vi "Calibration Helper.vi"(6 "Std Devs":cluster{"H":dbl, "S":dbl, "V":dbl}={"H"=4.0, "S"=6.0, "V"=4.0}, 8 "Color Mode":u16(ring)=2 items=["RGB", "HSL", "HSV", "HSI", "CIE L*a*b*", "CIE XYZ"], 9 "Color Components":T1={"Hue"={110.0, 142.0}, "Sat"={138.0, 255.0}, "Val"={139.0, 198.0}} {"Val" scale=0.0..255.0; "Sat" scale=0.0..255.0; "Hue" scale=0.0..255.0 scale format="%#_3g"}, 10 "Image":T2, 11 "Image Ctl Refnum":refnum<vi>) -> (2 "Changed":bool, 3 "output color":T3)   [LabVIEW 2025]
doc: "Process mouse clicks on the image control to compute a color range that describes the highlighted region. The range is based on the center and standard deviation returned by a histogram of the region."
uses:
  <vilib>/vision/Image Controls.llb/IMAQ Image.ctl
  <vilib>/vision/NI_Vision_Development_Module.lvlib
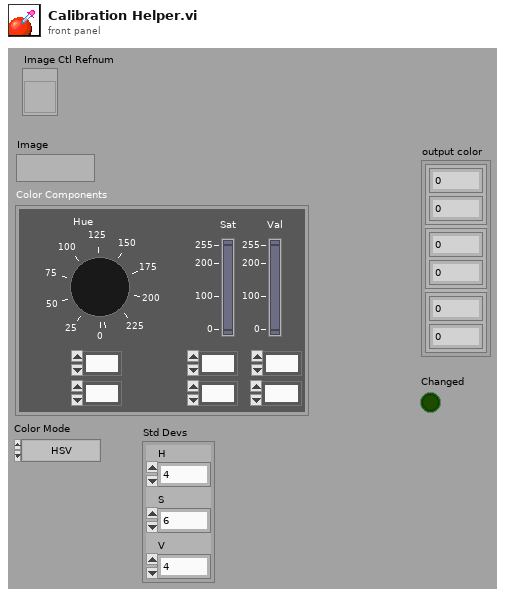
[diagram p1: front panel]
types:
  T1 = cluster{"Hue":cluster{dbl, dbl}, "Sat":cluster{dbl, dbl}, "Val":cluster{dbl, dbl}}
  T2 = typedef "IMAQ Image.ctl" = refnum<image>
  T3 = cluster{cluster{dbl, dbl}, cluster{dbl, dbl}, cluster{dbl, dbl}}
  T4 = typedef "Image Type" = u32
  T5 = cluster{"Global Rectangle":i32[], "Contours":cluster{"Contour Type":u32, "ROI Type":u32, "Points":i32[]}[]}
  T6 = cluster{"histogram":u32[], "Minimal Value":sgl, "Maximal Value":sgl, "Starting Value":sgl, "Interval Width":sgl, "Mean Value":sgl, "Standard  Variation":sgl, "Area (pixels)":i32}
  T7 = cluster{"histogram":u32[], "Minimal Value":sgl, "Maximal Value":sgl, "Starting Value":sgl, "Interval Width":sgl, "Mean Value":sgl, "Standard  Variation":sgl, "Area (pixels)":i32}[]
  T8 = cluster{"[0]":cluster{dbl, dbl}, "[1]":cluster{dbl, dbl}, "[2]":cluster{dbl, dbl}}
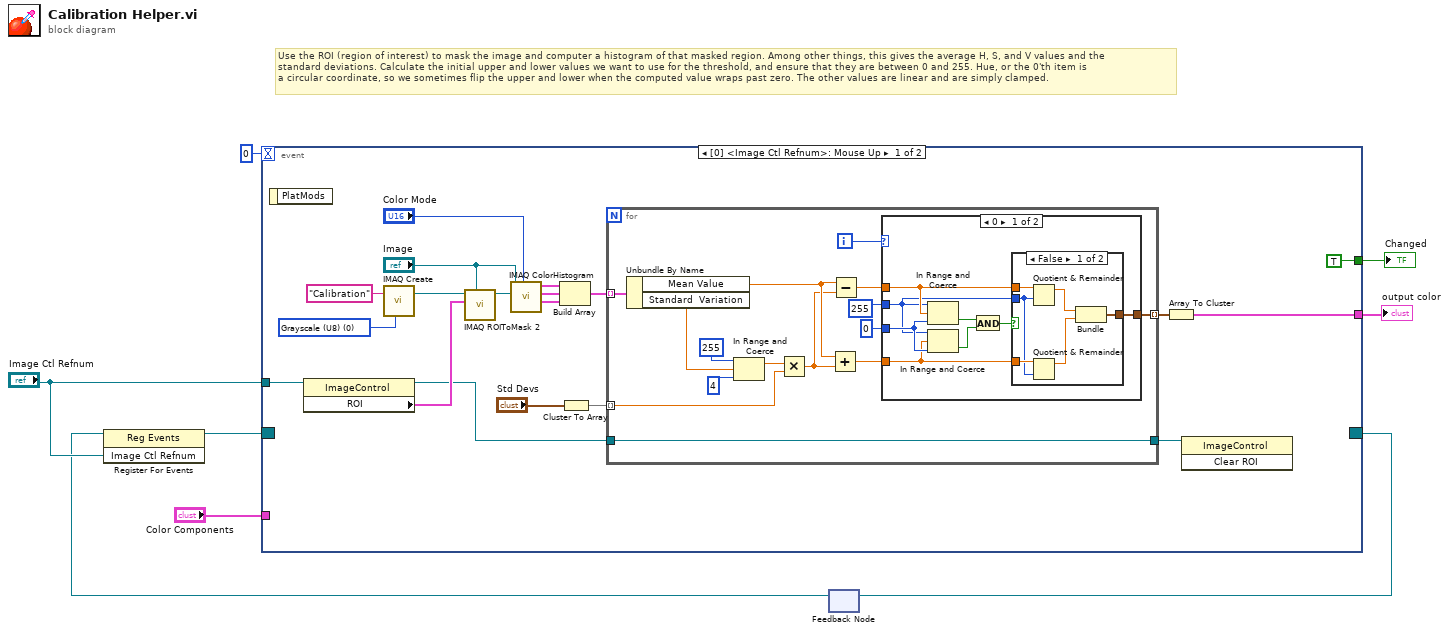
[diagram p0: block diagram]
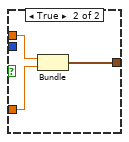
[diagram p2: hidden frame]
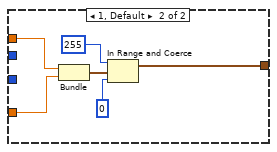
[diagram p3: hidden frame]
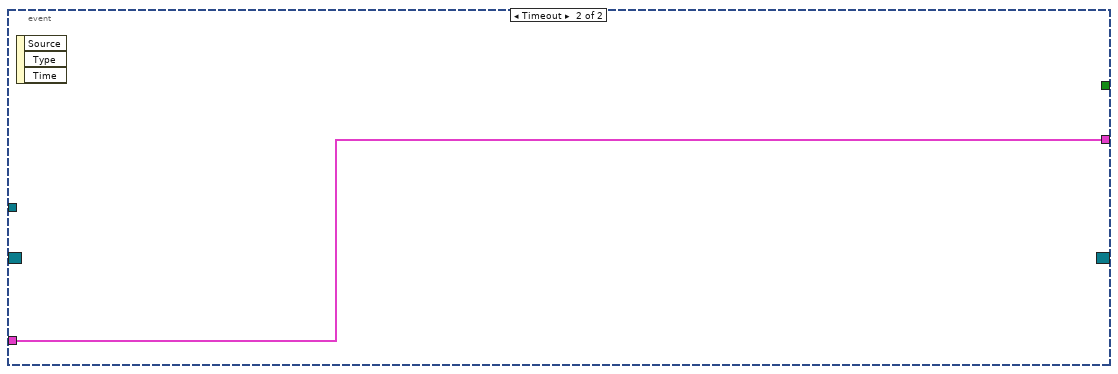
[diagram p4: hidden frame]
diagram:
  # "Use the ROI (region of interest) to mask the image and computer a histogram of that masked region. Among other things, this gives the average H, S, and V values and the\nstandard deviations. Calculate the initial upper and lower values we want to use for the threshold, and ensure that they are between 0 and 255. Hue, or the 0'th item is\na circular coordinate, so we sometimes flip the upper and lower when the computed value wraps past zero. The other values are linear and are simply clamped."
  n1 = feedback #1() -> (w2:refnum<event-registration>)  [unwired: 1 in]
  n2 = register-events(reference=w2, "Image Ctl Refnum") -> (reference out=w6:refnum<event-registration>)  [unwired: 1 in, 1 out]
  n3 = event shown="[0] <Image Ctl Refnum>: Mouse Up" {
    selector: w6 -> [_ _]
    dyn-events: [_ _] -> w3
    timeout: 0 -> [_ _]
    tunnel: "Image Ctl Refnum" -> [w14 _]
    tunnel: "Color Components" -> [_ w66]
    tunnel: [w10 w66] -> w4
    tunnel: [TRUE _] -> w1
    event Mouse Up {
      w27 = T4 0 items=["Grayscale (U8)", "Grayscale (I16)", "Grayscale (SGL)", "Complex (CSG)", "RGB (U32)", "HSL (U32)", "RGB (U64)", "Grayscale (U16)"] ("Image Type")
      n4 = event-data() -> ()  [unwired: 1 in, 1 out]
      n5 = property on="Property Node" class="ImageControl"(reference=w14) -> (reference out=w11:refnum<vi>, "ROI"=w13:T5)  [unwired: 1 in, 1 out]
      n6 = call "IMAQ Create"("Image Name"="Calibration", "Image Type"=w27) -> ("New Image"=w24:T2)  [unwired: 3 in, 1 out]
      n7 = call "IMAQ ROIToMask 2"("Image Model"="Image", "ROI Descriptor"=w13, "Image"=w24) -> ("Image Out"=w25:T2)  [unwired: 6 in, 2 out]
      n8 = call "IMAQ ColorHistogram"("Color Mode"="Color Mode", "Image Src"="Image", "Image Mask"=w25) -> ("Red or Hue or X or L* Histogram Report"=w20:T6, "Green or Sat or Y or a* Histogram Report"=w19:T6, "Blue or Luma or Val or Inten or Z or b* Histogram Report"=w18:T6)  [unwired: 3 in, 1 out]
      n9 = Build Array(w20, w19, w18) -> (w16:T7)
      n10 = Cluster To Array(cluster="Std Devs") -> (array=w17:dbl[])
      n11 = for {
        tunnel: w17 -> [w38] mode=indexing
        tunnel: w16 -> [w42] mode=indexing
        tunnel: [w33] -> w15 mode=indexing
        tunnel: [w28] -> w12
        tunnel: w11 -> [w28]
        i -> [w31]
        n12 = Unbundle By Name(w42) -> ("Mean Value"=w36:sgl, "Standard  Variation"=w39:sgl)
        n13 = In Range and Coerce(upper limit=255, x=w39, lower limit=4) -> (coerced(x)=w37:sgl)  [unwired: 1 out]
        n14 = Multiply(x=w37, y=w38) -> (x*y=w32:dbl)
        n15 = Add(x=w36, y=w32) -> (x+y=w34:dbl)
        n16 = Subtract(x=w36, y=w32) -> (x-y=w35:dbl)
        n17 = case shown="0" w31 {
          tunnel: w35 -> [w45 w62]
          tunnel: w34 -> [w44 w61]
          tunnel: [w47 w60] -> w33
          tunnel: 255 -> [w43 _]
          tunnel: 0 -> [w46 _]
          frame 0 {
            n18 = In Range and Coerce(upper limit=w43, x=w45, lower limit=w46) -> (In Range?=w49:bool)  [unwired: 1 out]
            n19 = In Range and Coerce(upper limit=w43, x=w44, lower limit=w46) -> (In Range?=w48:bool)  [unwired: 1 out]
            n20 = And(x=w49, y=w48) -> (x .and. y?=w50:bool)
            n21 = case shown="False" w50 {
              tunnel: [w53 w59] -> w47
              tunnel: w45 -> [w56 w57]
              tunnel: w44 -> [w55 w58]
              tunnel: w43 -> [w54 _]
              frame False {
                n22 = Quotient & Remainder(x=w56, y=w54) -> (x-y*floor(x/y)=w51:dbl)  [unwired: 1 out]
                n23 = Quotient & Remainder(x=w55, y=w54) -> (x-y*floor(x/y)=w52:dbl)  [unwired: 1 out]
                n24 = Bundle(w51, w52) -> (w53:cluster{dbl, dbl})  [unwired: 1 in]
              }
              frame True {
                n25 = Bundle(w57, w58) -> (w59:cluster{dbl, dbl})  [unwired: 1 in]
              }
            }
          }
          frame 1, Default {
            n26 = Bundle(w62, w61) -> (w65:cluster{dbl, dbl})  [unwired: 1 in]
            n27 = In Range and Coerce(upper limit=255, x=w65, lower limit=0) -> (coerced(x)=w60:cluster{dbl, dbl})  [unwired: 1 out]
          }
        }
      }
      n28 = Array To Cluster(array=w15) -> (cluster=w10:T8)
      n29 = invoke on="Invoke Node" class="ImageControl" method="Clear ROI"(reference=w12) -> ()  [unwired: 2 in, 3 out]
    }
    event Timeout {
      n30 = event-data() -> ()  [unwired: 1 in, 3 out]
    }
  }
  "output color" <- w4
  "Changed" <- w1
  n31 = feedback-in #1(w3) -> ()
